vi "ITjsonOut.vi"(8 "error in (no error)":errorcluster, 11 "Data In":T1) -> (0 "error out":errorcluster, 3 "Data Out":T1)   [LabVIEW 2014]
uses:
  controls/Data1.ctl
  controls/Payjson.ctl
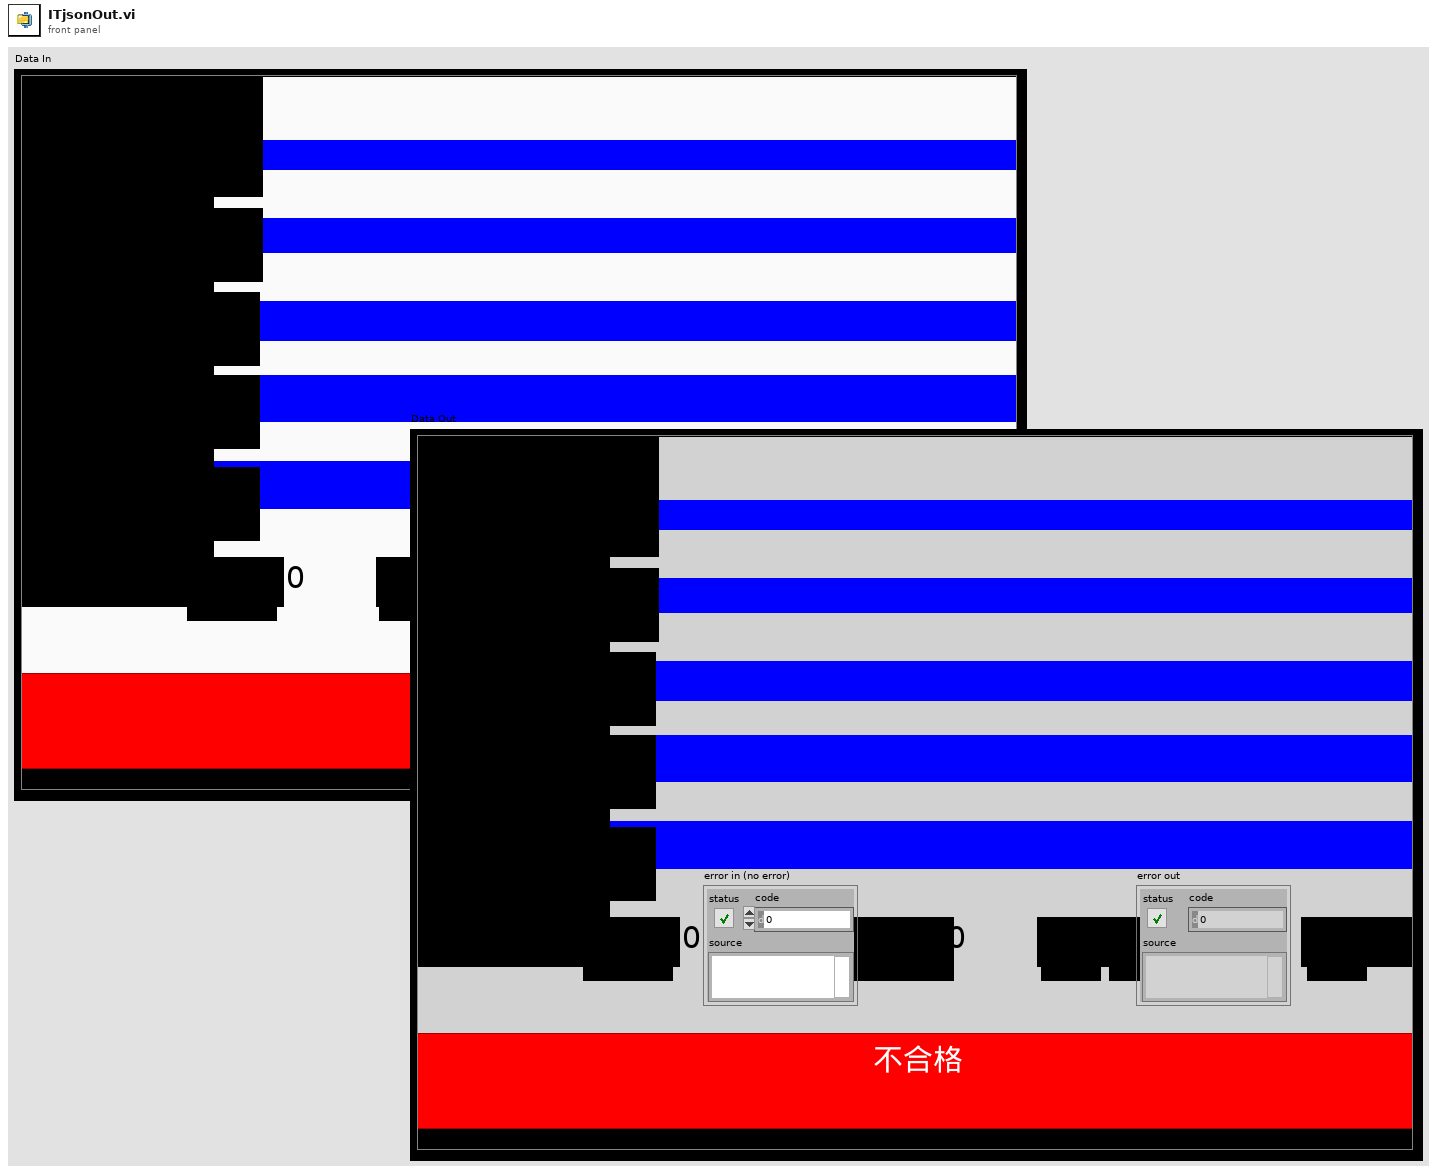
[diagram p1: front panel]
types:
  T1 = typedef "Data1.ctl" = cluster{"Date":string, "BarCode1":string, "BarCode2":string, "BarCode3":string, "Message":string, "OK Count":u16, "NG Count":u16, "Total Count":u16, "ModelData":string[][], "OK&NG":bool, "COM1":refnum<visa-resource-name>, "COM2":refnum<visa-resource-name>, "IO":i32, "Time":u32, "TCP":refnum<k5>, "TCP 2":refnum<k5>, "COM1 2":refnum<visa-resource-name>, "CheckNum":string, "BarCode1_1":string, "BarCode2_1":string, "BarCode3_1":string, "日期":string, "機種":string, "機號":string, "商品條碼1":string, "OK_1":string, "OK":string, "NG":string, "NG_1":string, "Total":string, "Total_1":string, "ClaerTime":u32, "Pjson":T2, "LotNo":string[], "CheckParsArray":string[], "BarCode4":string, "BarCode4_1":string, "商品條碼2":string, "BarCode5":string, "BarCode5_1":string, "商品條碼3":string, "ReScanNG":i32, "NGTimeCT":u32}
  T2 = typedef "Payjson.ctl" = cluster{"DEPT":string, "LINE":string, "STANO":string, "WORKNO":string, "PRODSN":string, "COMPNTID":string, "COMPNTLOT":string, "COMPNTSN":string, "USEDQTY":i16, "OPDATE":string, "OPUSER":string, "RECVDATE":string, "MMODU":string}[]
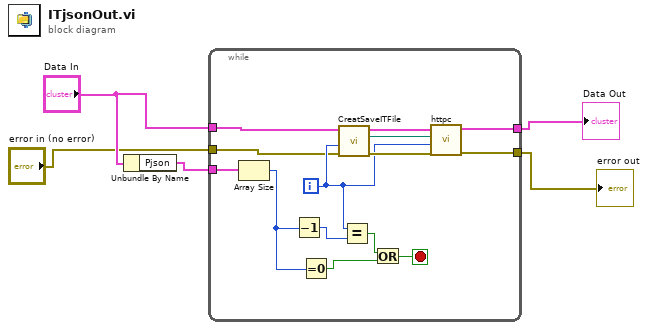
[diagram p0: block diagram]
diagram:
  n1 = Unbundle By Name("Data In") -> ("Pjson"=w4:T2)
  n2 = while {
    tunnel: "Data In" -> [w16]
    tunnel: w4 -> [w15]
    tunnel: [w8] -> w3
    tunnel: [w7] -> w1
    tunnel: "error in (no error)" -> [w6]
    i -> [w14]
    stop <- w9 stop-if-true
    n3 = Array Size(array=w15) -> (size(s)=w11:i32)
    n4 = Decrement(x=w11) -> (x-1=w13:i32)
    n5 = Equal To 0?(x=w11) -> (x = 0?=w10:bool)
    n6 = call "CreatSaveITFile.vi"("error in (no error)"=w6, "index"=w14, "Data in"=w16) -> ("error out"=w19:errorcluster, "ITFileSave path"=w17:path, "Data out"=w18:T1)  [unwired: 6 in]
    n7 = Equal?(x=w14, y=w13) -> (x = y?=w12:bool)
    n8 = Or(x=w12, y=w10) -> (x .or. y?=w9:bool)
    n9 = call "httpc.vi"("error in (no error)"=w19, "index"=w14, "ITFileSave path"=w17, "Data_in"=w18) -> ("error out"=w7:errorcluster, "Data_out"=w8:T1)  [unwired: 6 in]
  }
  "Data Out" <- w3
  "error out" <- w1
